vi "S2C_FORNAX_Proc_Status.vi"(8 "Error In":errorcluster) -> (0 "Error Out":errorcluster, 3 "Response":string)   [LabVIEW 2015]
uses:
  S2C_FORNAX_Proc_Globals.vi
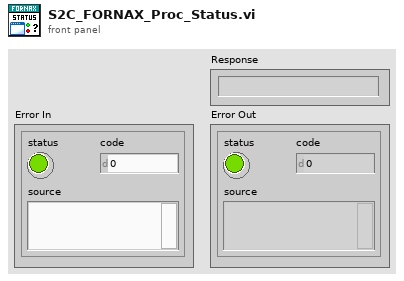
[diagram p1: front panel]
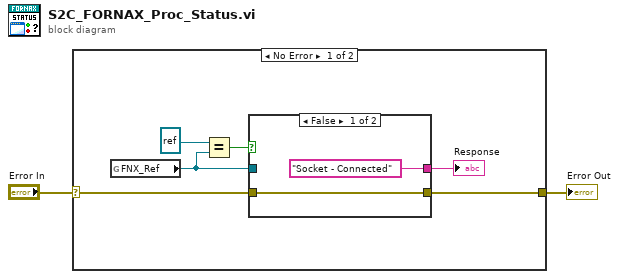
[diagram p0: block diagram]
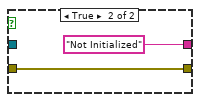
[diagram p2: hidden frame]
diagram:
  n1 = case shown="No Error" "Error In" {
    selector: "Error In" -> [w8 w13]
    tunnel: [w7 w13] -> w1
    frame No Error {
      n2 = global read "S2C_FORNAX_Proc_Globals.vi" "FNX_Ref"() -> (w4:refnum<k5>)
      n3 = Equal?(x=refnum<k5> refnum ("5190-Tcp"), y=w4) -> (x = y?=w3:bool)
      n4 = case shown="False" w3 {
        tunnel: w8 -> [w10 w12]
        tunnel: w4 -> [_ _]
        tunnel: [w10 w12] -> w7
        tunnel: ["Socket - Connected" "Not Initialized" ("f")] -> w6
        frame False {
        }
        frame True {
        }
      }
      "Response" <- w6
    }
    frame Error {
    }
  }
  "Error Out" <- w1
